vi "Transmit-message.vi"(8 "error in (no error)":errorcluster, 10 "Message":refnum<class "Message.lvclass">, 11 "ModComm in":T1) -> (0 "error out":errorcluster, 3 "ModComm out":T1)   [LabVIEW 2013, in "Server.lvlib" / "Server.lvclass"]
uses:
  Server.lvclass
  Object-reference.ctl
  Messages/Sources/Message.lvclass
  Messages/Sources/Message.lvclass/Message.ctl
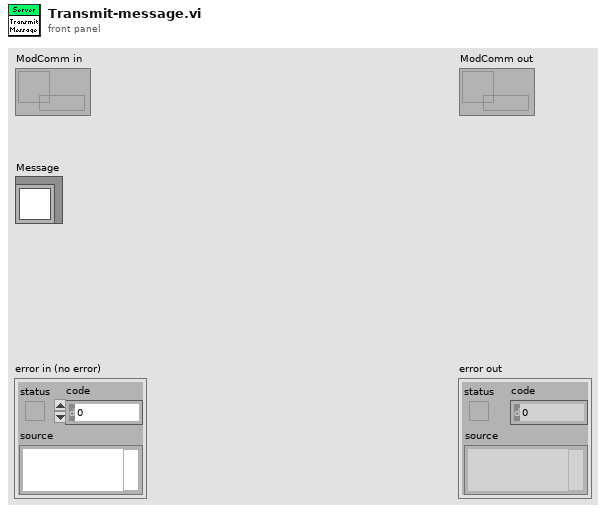
[diagram p1: front panel]
types:
  T1 = typedef "Server.lvlib/Server.lvclass/Object-reference.ctl" = refnum<data-value>
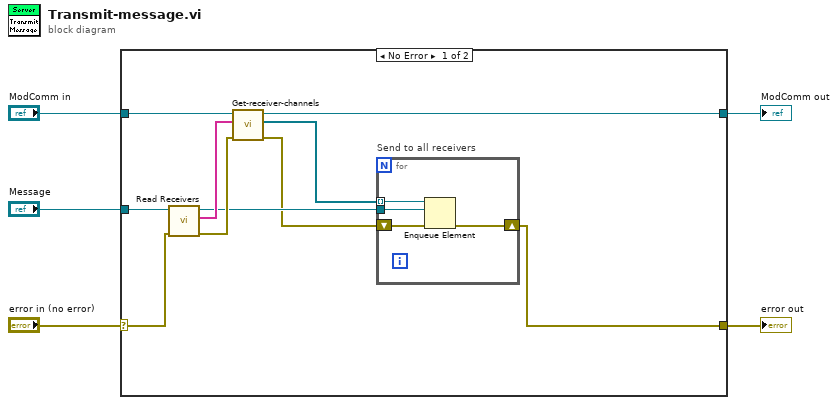
[diagram p0: block diagram]
diagram:
  n1 = case shown="No Error" "error in (no error)" {
    selector: "error in (no error)" -> [w7 w21]
    tunnel: [w6 w21] -> w4
    tunnel: [w14 w20] -> w2
    tunnel: "ModComm in" -> [w15 w20]
    tunnel: "Message" -> [w13 _]
    frame No Error {
      n2 = call "Read Receivers.vi"("error in (no error)"=w7, "Message in"=w13) -> ("error out"=w11:errorcluster, "Receivers"=w12:string[], "Message out"=w10:refnum<class "Message.lvclass">)  [unwired: 7 in]
      n3 = call "Get-receiver-channels.vi"("error in (no error)"=w11, "Receivers"=w12, "ModComm in"=w15) -> ("error out"=w9:errorcluster, "Receiver channels"=w8:refnum<queue>[], "ModComm out"=w14:T1)  [unwired: 6 in]
      n4 = for "Send to all receivers" {
        tunnel: w10 -> [w18]
        tunnel: w8 -> [w16] mode=indexing
        shift-right: [w19] -> w6
        shift-left: w9 -> [w17]
        n5 = Enqueue Element(queue=w16, element=w18, error in (no error)=w17) -> (error out=w19:errorcluster)  [unwired: 1 in, 2 out]
      }
    }
    frame Error {
    }
  }
  "error out" <- w4
  "ModComm out" <- w2
